vi "CheckPump.vi"(7 "ValidCh":T3[](array[typedef]) items=["7"=7, "11"=11, "12"=12, "13"=13, "15"=15, "16"=16, "18"=18, "29"=29, "32"=32, "33"=33, "35"=35, "36"=36, "37"=37, "38"=38, "40"=40], 8 "error in":errorcluster, 9 "Channel No in":T3=29 items=["7"=7, "11"=11, "12"=12, "13"=13, "15"=15, "16"=16, "18"=18, "29"=29, "32"=32, "33"=33, "35"=35, "36"=36, "37"=37, "38"=38, "40"=40], 10 "PI_REF":T4, 11 "Read_Write_Valv_IN":T1 {"ValidCh" items=["7"=7, "11"=11, "12"=12, "13"=13, "15"=15, "16"=16, "18"=18, "29"=29, "32"=32, "33"=33, "35"=35, "36"=36, "37"=37, "38"=38, "40"=40]}) -> (0 "error out":errorcluster, 3 "Read_Write_Valv_OUT":T1 {"ValidCh" items=["7"=7, "11"=11, "12"=12, "13"=13, "15"=15, "16"=16, "18"=18, "29"=29, "32"=32, "33"=33, "35"=35, "36"=36, "37"=37, "38"=38, "40"=40]})   [LabVIEW 2014, in "ValveCTRL.lvlib"]
uses:
  ValveCTRL.lvlib
  TypeDef/CHs_List.ctl
  <vilib>/MakerHub/LINX/Private/Type Defs/LINX Ref.ctl
  <vilib>/MakerHub/LINX/Private/Type Defs/Platform.ctl
  <vilib>/MakerHub/LINX/Private/Type Defs/Interface.ctl
  <vilib>/MakerHub/LINX/Private/Device/Type Defs/LINX Device Config.ctl
  <vilib>/MakerHub/LINX/Private/Device/Type Defs/TCP Config.ctl
  <vilib>/MakerHub/LINX/Private/Device/Type Defs/Channels.ctl
  TypeDef/Read_Write.ctl
  TypeDef/ChannelStatus.ctl
  <vilib>/Utility/error.llb/Error Cluster From Error Code.vi
  <vilib>/ErrorRing/Error Ring.xnode
  Main/Main.lvlib
  <vilib>/MakerHub/LINX/LMH-LINX.lvlib
  <vilib>/MakerHub/LINX/Private/Device/Device.lvlib
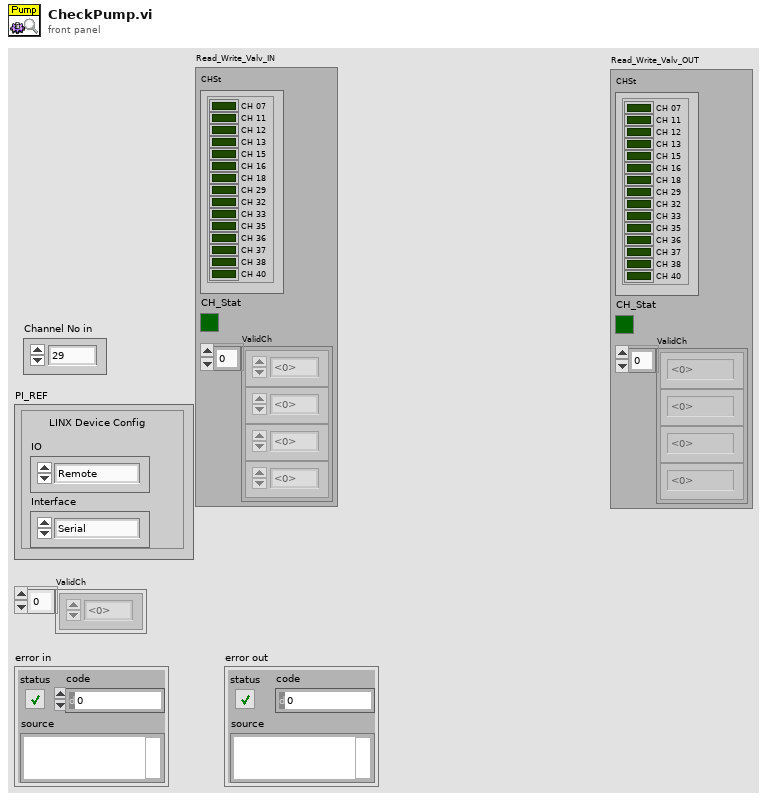
[diagram p1: front panel]
types:
  T1 = typedef "ValveCTRL.lvlib/Read_Write.ctl" = cluster{"CHSt":T2, "CH_Stat":bool, "ValidCh":T3[]}
  T2 = typedef "ValveCTRL.lvlib/ChannelStatus.ctl" = cluster{"CH 07":bool, "CH 11":bool, "CH 12":bool, "CH 13":bool, "CH 15":bool, "CH 16":bool, "CH 18":bool, "CH 29":bool, "CH 32":bool, "CH 33":bool, "CH 35":bool, "CH 36":bool, "CH 37":bool, "CH 38":bool, "CH 40":bool}
  T3 = typedef "ValveCTRL.lvlib/CHs_List.ctl" = u8
  T4 = typedef "LMH-LINX.lvlib/LINX Ref.ctl" = cluster{"IO":T5, "Interface":T6, "LINX Device Config":T7}
  T5 = typedef "LMH-LINX.lvlib/Platform.ctl" = enum16{"Remote", "Local"}
  T6 = typedef "LMH-LINX.lvlib/Interface.ctl" = enum16{"Serial", "TCP"}
  T7 = typedef "LMH-LINX.lvlib/Device.lvlib/LINX Device Config.ctl" = cluster{"Interface":T6, "COM Port":refnum<visa-resource-name>, "TCP Configuration":T8, "Device Family":u8, "Device ID":u8, "Device Name":string, "TCP Ref":refnum<k5>, "Channels":T9}
  T8 = typedef "LMH-LINX.lvlib/Device.lvlib/TCP Config.ctl" = cluster{"IP Address":string, "Port":u16}
  T9 = typedef "LMH-LINX.lvlib/Channels.ctl" = cluster{"DI":u8[], "DO":u8[], "AI":u8[], "AO":u8[], "PWM":u8[], "QE":u8[], "UART":u8[], "I2C 2":u8[], "SPI":u8[], "CAN":u8[], "Servo":u8[], "AI Ref (V)":dbl, "AI Resolution (Bits)":u8, "AO Ref (V)":dbl, "AO Resolution (Bits)":u8}
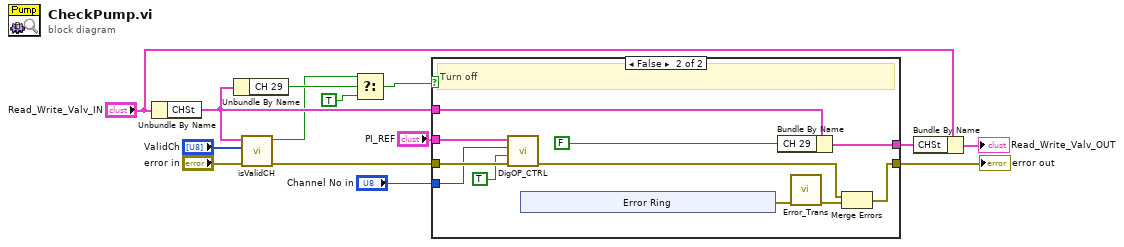
[diagram p0: block diagram]
diagram:
  n1 = Unbundle By Name("Read_Write_Valv_IN") -> ("CHSt"=w8:T2)
  n2 = Unbundle By Name(w8) -> ("CH 29"=w4:bool)
  n3 = call "isValidCH.vi"("error in"="error in", "ValidCh"="ValidCh", "CHStIn"=w8) -> ("error out"=w10:errorcluster, "VaildCH?"=w3:bool)  [unwired: 7 in]
  n4 = Select(t=w3, s=w4, f=TRUE) -> (s? t:f=w2:bool)
  n5 = case shown="False" w2 {
    tunnel: [w16 w17] -> w12
    tunnel: w10 -> [w16 w27]
    tunnel: "Channel No in" -> [_ w25]
    tunnel: "PI_REF" -> [_ w24]
    tunnel: w8 -> [w15 w23]
    tunnel: [w15 w22] -> w6
    frame True {
      # "Do not change the state"
    }
    frame False {
      # "Turn off"
      n6 = call "DigOP_CTRL.vi"("Error In"=w27, "Output Value"=TRUE, "Channel No"=w25, "LINX Resource In"=w24) -> ("Error Out"=w18:errorcluster)  [unwired: 5 in, 2 out]
      n7 = xnode "Error Ring"() -> ("error out"=w20:errorcluster)
      n8 = Bundle By Name(cluster=w23, "CH 29"=FALSE ("Output Value")) -> (w22:T2)
      n9 = call "Error_Trans.vi"("Error In"=w20) -> ("Error Out"=w19:errorcluster)  [unwired: 9 in, 1 out]
      n10 = Merge Errors(w18, w19) -> (w17:errorcluster)
    }
  }
  "error out" <- w12
  n11 = Bundle By Name(cluster="Read_Write_Valv_IN", "CHSt"=w6) -> (→"Read_Write_Valv_OUT":T1)
